vi "Prepare - Load and Apply Window Settings.vi"(7 "This VI":refnum<vi>, 8 "error in (no error)":errorcluster, 11 "hse-config":refnum<class "config-base.lvclass">) -> (0 "error out":errorcluster)   [LabVIEW 2022 SP3, in "UI Manager.lvlib"]
doc: "____\nHAMPEL SOFTWARE ENGINEERING v2.6.0 (2023-12-19 10:54)"
uses:
  UI Manager.lvlib
  Libraries/hse-libraries/Source/hse-configuration/config-base/config-base.lvclass
  <vilib>/Utility/miscctls.llb/LVRectTypeDef.ctl
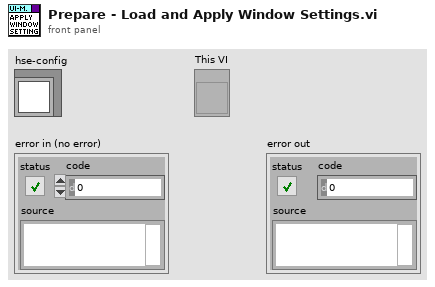
[diagram p1: front panel]
types:
  T1 = cluster{"width":i16, "height":i16, "state":string, "monitor":u16, "closeable":bool, "show_runtimemenu":bool, "smooth_fade_in":bool, "resizeable":bool, "minimizable":bool}
  T2 = typedef "LVRectTypeDef.ctl" = cluster{"Left":i16, "Top":i16, "Right":i16, "Bottom":i16}
  T3 = typedef "LVPointTypeDef.ctl" = cluster{"Horizontal":i16, "Vertical":i16}
  T4 = enum32{"Invalid", "Standard", "Closed", "Hidden", "Minimized", "Maximized"}
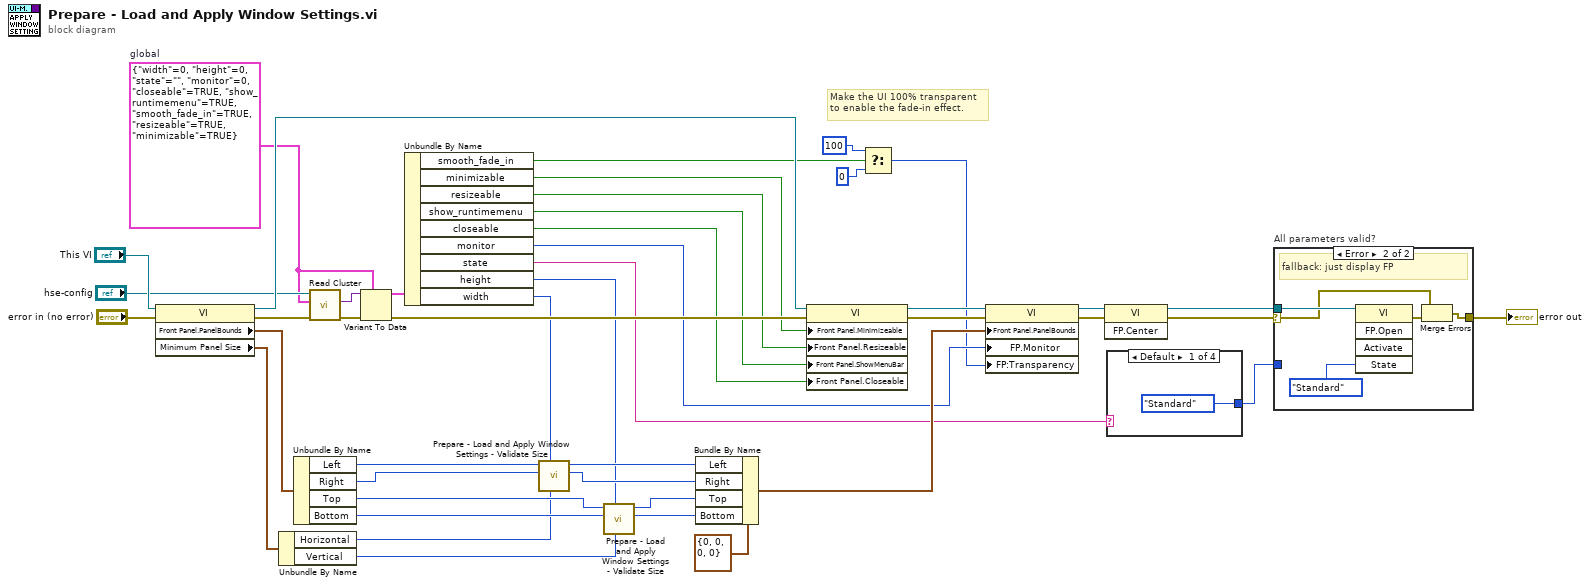
[diagram p0: block diagram]
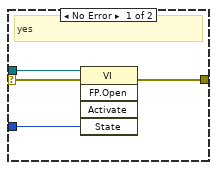
[diagram p2: hidden frame]
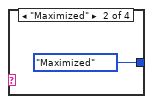
[diagram p3: hidden frame]
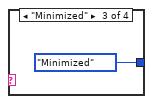
[diagram p4: hidden frame]
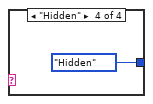
[diagram p5: hidden frame]
diagram:
  w15 = T1 {"width"=0, "height"=0, "state"="", "monitor"=0, "closeable"=TRUE, "show_runtimemenu"=TRUE, "smooth_fade_in"=TRUE, "resizeable"=TRUE, "minimizable"=TRUE}  # global
  # "Make the UI 100% transparent\nto enable the fade-in effect."
  n1 = property class="VI"(reference="This VI", error in="error in (no error)") -> (reference out=w36:refnum<vi>, error out=w19:errorcluster, "Front Panel.PanelBounds"=w35:T2, "Minimum Panel Size"=w25:T3)
  n2 = Unbundle By Name(w25) -> ("Horizontal"=w24:i16, "Vertical"=w23:i16)
  n3 = Unbundle By Name(w35) -> ("Left"=w33:i16, "Right"=w32:i16, "Top"=w27:i16, "Bottom"=w29:i16)
  n4 = call-dynamic "Read Cluster.vi"("error in"=w19, "Type in"=w15, "config-base in"="hse-config") -> ("error out"=w17:errorcluster, "Value Cluster out"=w16:variant)  [unwired: 6 in, 1 out]
  n5 = Variant To Data(error in=w17, type=w15, Variant=w16) -> (data=w14:T1, error out=w13:errorcluster)
  n6 = Unbundle By Name(w14) -> ("smooth_fade_in"=w2:bool, "minimizable"=w1:bool, "resizeable"=w3:bool, "show_runtimemenu"=w7:bool, "closeable"=w8:bool, "monitor"=w9:u16, "state"=w10:string, "height"=w11:i16, "width"=w12:i16)
  n7 = call "Prepare - Load and Apply Window Settings - Validate Size.vi"("Minimum"=w24, "New Size"=w12, "Current Right/Bottom"=w32, "Current Left/Top"=w33) -> ("New Right/Bottom"=w30:i16, "New Left/Top"=w31:i16)  [unwired: 6 in]
  n8 = call "Prepare - Load and Apply Window Settings - Validate Size.vi"("Minimum"=w23, "New Size"=w11, "Current Right/Bottom"=w29, "Current Left/Top"=w27) -> ("New Right/Bottom"=w28:i16, "New Left/Top"=w26:i16)  [unwired: 6 in]
  n9 = Bundle By Name(cluster=T2 {"Left"=0, "Top"=0, "Right"=0, "Bottom"=0} ("Front Panel Window:Window Bounds"), "Left"=w31, "Right"=w30, "Top"=w26, "Bottom"=w28) -> (w42:T2)
  n10 = property class="VI"(reference=w36, error in=w13, "Front Panel.Minimizeable"=w1, "Front Panel.Resizeable"=w3, "Front Panel.ShowMenuBar"=w7, "Front Panel.Closeable"=w8) -> (reference out=w40:refnum<vi>, error out=w41:errorcluster)
  n11 = Select(t=u8 100 ("Front Panel Window:Transparency"), s=w2, f=u8 0) -> (s? t:f=w4:u8)
  n12 = property class="VI"(reference=w40, error in=w41, "Front Panel.PanelBounds"=w42, "FP.Monitor"=w9, "FP:Transparency"=w4) -> (reference out=w34:refnum<vi>, error out=w39:errorcluster)
  n13 = invoke class="VI" method="FP.Center"(reference=w34, error in=w39) -> (reference out=w21:refnum<vi>, error out=w20:errorcluster)  [unwired: 1 in, 1 out]
  n14 = case shown="Default" w10 {
    tunnel: [T4."Standard" ("State") T4."Maximized" ("State") T4."Minimized" ("State") T4."Hidden" ("State")] -> w44
    frame Default {
    }
    frame "Maximized" {
    }
    frame "Minimized" {
    }
    frame "Hidden" {
    }
  }
  n15 = case "All parameters valid?" shown="Error" w20 {
    selector: w20 -> [w50 w53]
    tunnel: w44 -> [w52 _]
    tunnel: w21 -> [w51 w57]
    tunnel: [w49 w54] -> w22
    frame No Error {
      # "yes"
      n16 = invoke class="VI" method="FP.Open"(reference=w51, error in=w50, "State"=w52) -> (error out=w49:errorcluster)  [unwired: 2 in, 4 out]
    }
    frame Error {
      # "fallback: just display FP"
      n17 = invoke class="VI" method="FP.Open"(reference=w57, "State"=T4."Standard") -> (error out=w56:errorcluster)  [unwired: 3 in, 4 out]
      n18 = Merge Errors(w53, w56) -> (w54:errorcluster)
    }
  }
  "error out" <- w22
